vi "CFTS-Open Vitals Monitor.vi"() -> (15 "error out":errorcluster)   [LabVIEW 2020]
uses:
  <vilib>/registry/registry.llb/Registry SAM.ctl
  <vilib>/registry/registry.llb/Registry View.ctl
  <vilib>/registry/registry.llb/Read Registry Value Simple STR.vi
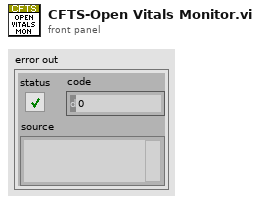
[diagram p1: front panel]
types:
  T1 = enum16{"big-endian, network order", "native, host order", "little-endian"}
  T2 = typedef "Registry SAM.ctl" = enum32{"KEY_QUERY_VALUE", "KEY_SET_VALUE", "KEY_CREATE_SUB_KEY", "KEY_ENUMERATE_SUB_KEYS", "KEY_NOTIFY", "KEY_CREATE_LINK", "KEY_READ", "KEY_WRITE", "KEY_ALL_ACCESS", "KEY_READ | KEY_WRITE"}
  T3 = typedef "Registry View.ctl" = u16
  T4 = typedef "Registry refnum.ctl" = refnum<k1>
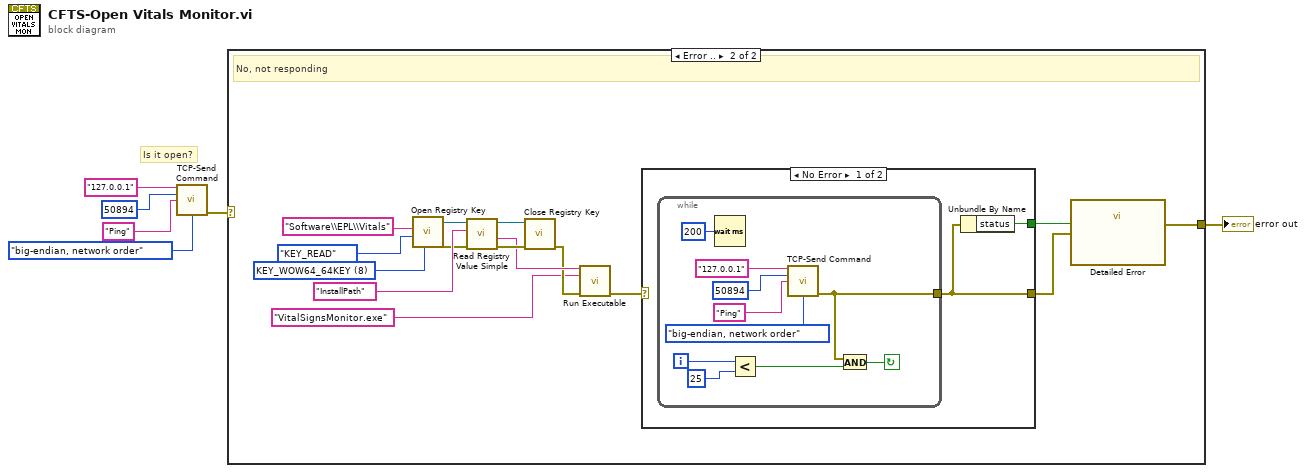
[diagram p0: block diagram]
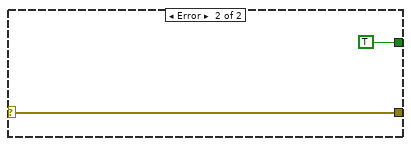
[diagram p3: hidden frame]
diagram:
  # "Is it open?"
  n1 = call "TCP-Send Command.vi"("PXI Address"="127.0.0.1", "Port"=50894, "Command"="Ping", "byte order"=T1."big-endian, network order") -> ("error out"=w3:errorcluster)  [unwired: 11 in]
  n2 = case shown="Error .." w3 {
    tunnel: [_ w21] -> w2
    frame No Error {
      # "Yes, it's open"
    }
    frame Error {
      w15 = T3 8 items=["Default"=0, "KEY_WOW64_64KEY"=8, "KEY_WOW64_32KEY"=9] ("registry view")
      # "No, not responding"
      n3 = call <vilib>:"Open Registry Key.vi"("registry view"=w15, "security access mask (KEY_READ | KEY_WRITE)"=Registry_SAM."KEY_READ", "subkey"="Software\\EPL\\Vitals") -> ("error out"=w17:errorcluster, "refnum out"=w19:T4)  [unwired: 7 in]
      n4 = call-poly <vilib>:"Read Registry Value Simple.vi"("error in (no error)"=w17, "value"="InstallPath", "refnum"=w19) -> ("error out"=w14:errorcluster, "String/Binary data"=w12:string, "refnum out"=w13:T4)  [unwired: 3 in, 1 out]
      n5 = call <vilib>:"Close Registry Key.vi"("error in (no error)"=w14, "refnum"=w13) -> ("error out"=w11:errorcluster)  [unwired: 5 in]
      n6 = call "Run Executable.vi"("Folder"=w12, ".EXE name"="VitalSignsMonitor.exe" ("value"), "error in (no error)"=w11) -> ("error out"=w9:errorcluster)  [unwired: 12 in]
      n7 = case shown="No Error" w9 {
        selector: w9 -> [_ w35]
        tunnel: [w22 w35] -> w8
        tunnel: [w23 TRUE ("Error?")] -> w7
        frame No Error {
          n8 = while {
            tunnel: [w25] -> w22
            i -> [w29]
            stop <- w26 continue-if-true
            n9 = Wait (ms)(milliseconds to wait=u32 200) -> ()  [unwired: 1 out]
            n10 = Less?(x=w29, y=25) -> (x < y?=w27:bool)
            n11 = call "TCP-Send Command.vi"("PXI Address"="127.0.0.1", "Port"=50894, "Command"="Ping", "byte order"=T1."big-endian, network order") -> ("error out"=w25:errorcluster)  [unwired: 11 in]
            n12 = And(x=w25, y=w27) -> (x .and. y?=w26:bool)
          }
          n13 = Unbundle By Name(w22) -> ("status"=w23:bool)
        }
        frame Error {
        }
      }
      n14 = call "Detailed Error"("Error?"=w7, "Primary"=w8) -> ("detailed error"=w21:errorcluster)  [unwired: 13 in]
    }
  }
  "error out" <- w2
